vi "Preview Byte At Index.vi"(8 "error in (no error)":errorcluster, 9 "index (-1: last)":i32=-1, 11 "ByteFIFO":refnum<data-value>) -> (0 "error out":errorcluster, 1 "found":bool, 2 "byte":u8 format="%02x", 3 "ByteFIFO":refnum<data-value>)   [LabVIEW 2013, in "CircularBuffer.lvlib" / "ByteFIFO.lvclass"]
uses:
  ByteFIFO.lvclass
  VariantBuffer/VariantBuffer.lvclass
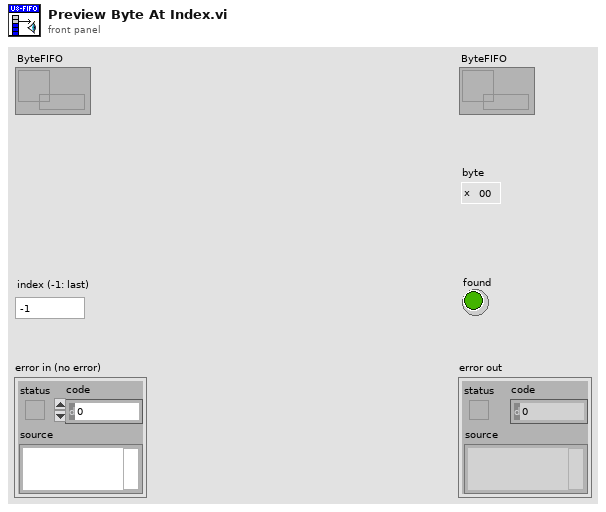
[diagram p1: front panel]
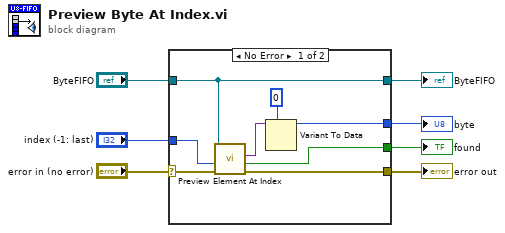
[diagram p0: block diagram]
diagram:
  n1 = case shown="No Error" "error in (no error)" {
    selector: "error in (no error)" -> [w14 w17]
    tunnel: [w10 w17] -> w6
    tunnel: [w15 w16] -> w4
    tunnel: "ByteFIFO" -> [w15 w16]
    tunnel: [w11 _] -> w3
    tunnel: [w8 _] -> w2
    tunnel: "index (-1: last)" -> [w9 _]
    frame No Error {
      n2 = call "Preview Element At Index.vi"("error in"=w14, "index (-1: last)"=w9, "Buffer in"=w15) -> ("error out"=w10:errorcluster, "found"=w8:bool, "element"=w13:variant)  [unwired: 5 in, 1 out]
      n3 = Variant To Data(type=u8 0 ("byte"), Variant=w13) -> (data=w11:u8)  [unwired: 1 in, 1 out]
    }
    frame Error {
    }
  }
  "error out" <- w6
  "ByteFIFO" <- w4
  "byte" <- w3
  "found" <- w2
